vi "DAQmx Run.vi"(11 "Shuwdown Event":refnum<user-event>) -> ()   [LabVIEW 2018, in "Hardware Control.lvlib"]
doc: "<b>Execution System:</b> Data Acquisition"
uses:
  Hardware Control.lvlib
  DAQmx Shortcut.ctl
  Messaging/Message Cluster.ctl
  <vilib>/DAQmx/read.llb/DAQmx Read (Digital 1D Bool NChan 1Samp 1Line).vi
  <vilib>/DAQmx/read.llb/DAQmx Read (Analog 2D DBL NChan NSamp).vi
  <vilib>/Analysis/baseanly.llb/Mean (DBL).vi
  <vilib>/DAQmx/miscellaneous.llb/DAQmx Fill In Error Info.vi
  <vilib>/DAQmx/configure/timing.llb/DAQmx Timing (Sample Clock).vi
  <resource>/objmgr/daqmx.rc
  Messaging/Messaging.lvlib
  <vilib>/Analysis/NI_AALBase.lvlib
panel:
  out "DI Error":errorcluster
  out "AI Error":errorcluster
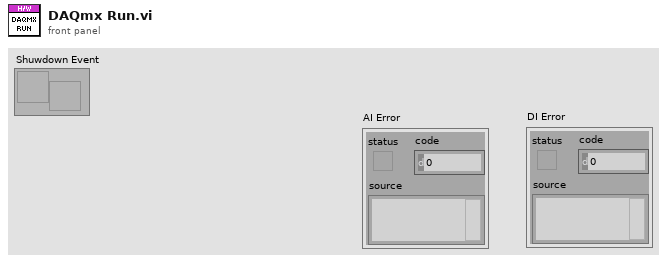
[diagram p1: front panel]
types:
  T1 = typedef "Hardware Control.lvlib/DAQmx Shortcut.ctl" = cluster{"DAQmx Global Channel":refnum<k21>, "Message Queue":string, "Event":string, "Target":string, "Data":variant}
  T2 = typedef "Messaging.lvlib/Message Cluster.ctl" = cluster{"Event":string, "Source":string, "Target":string, "Data":variant}
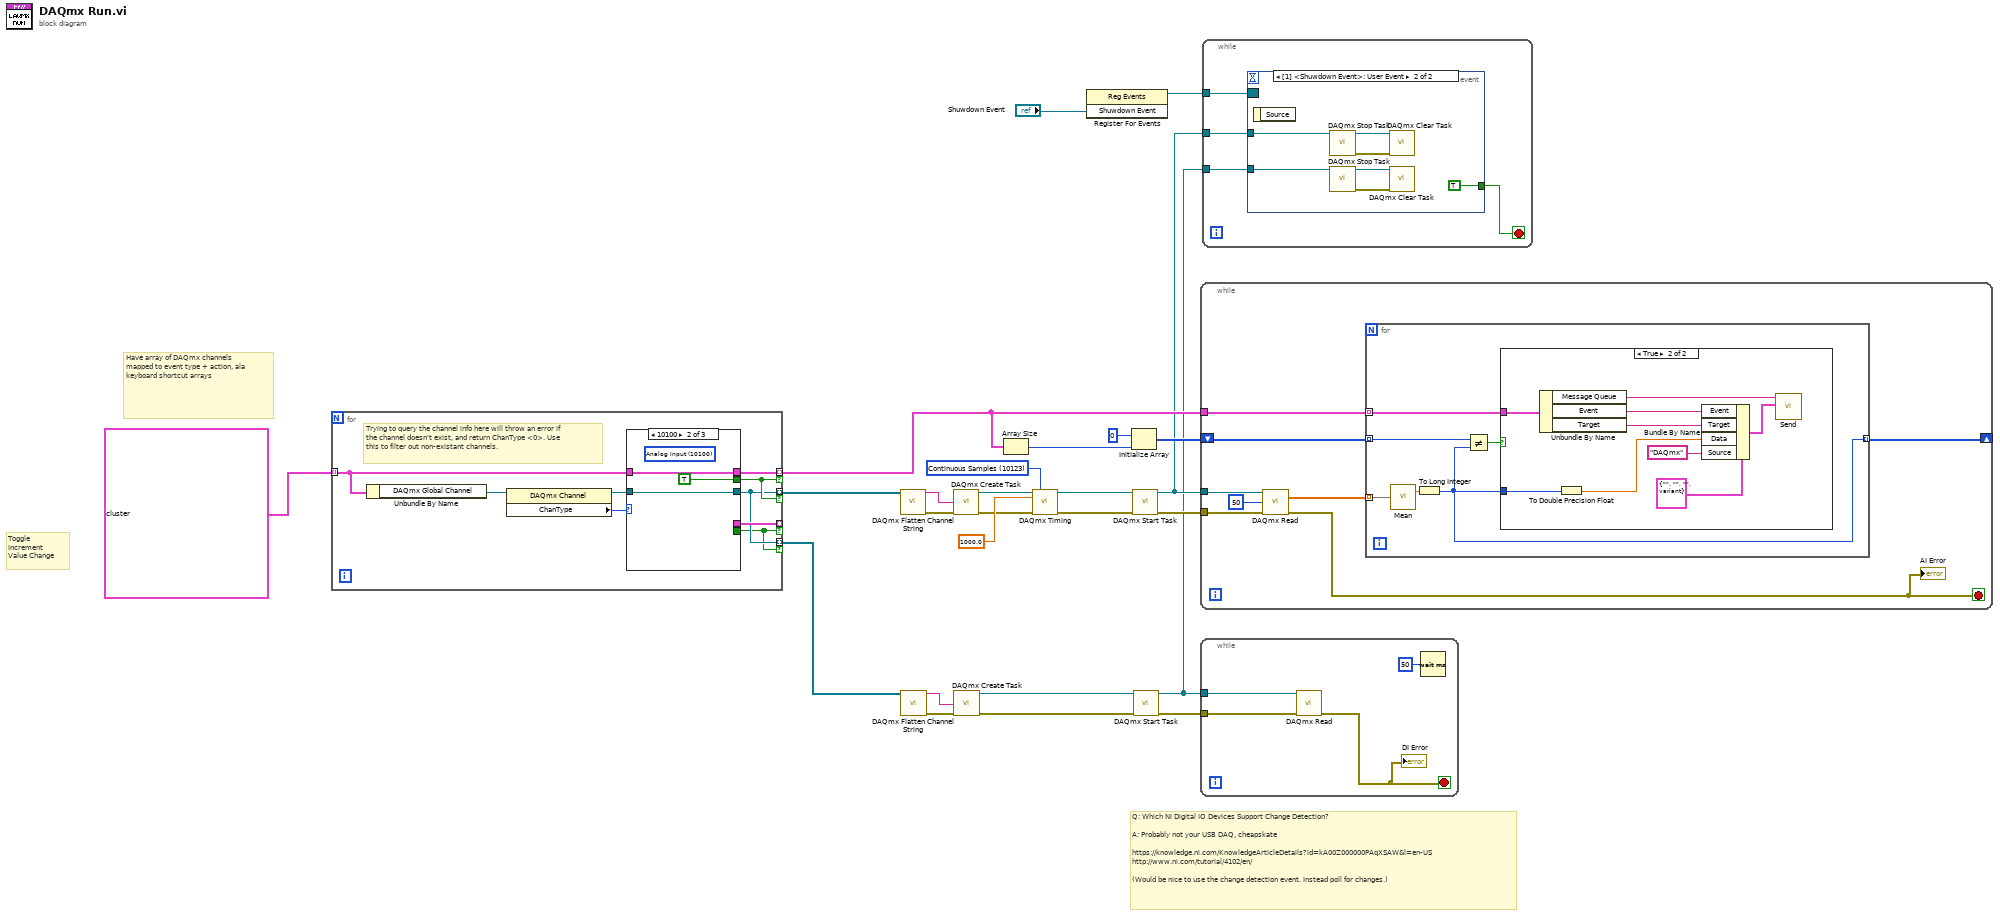
[diagram p0: block diagram]
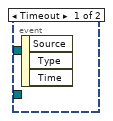
[diagram p2: hidden frame]
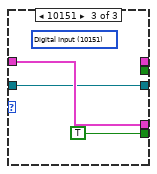
[diagram p5: hidden frame]
diagram:
  w24 = 10123 items=["Finite Samples"=10178, "Continuous Samples"=10123, "Hardware Timed Single Point"=12522] ("sample mode")
  # "Toggle\nIncrement\nValue Change"
  # "Have array of DAQmx channels mapped to event type + action, ala keyboard shortcut arrays"
  # "Q: Which NI Digital IO Devices Support Change Detection?\n\nA: Probably not your USB DAQ, cheapskate\n\nhttps://knowledge.ni.com/KnowledgeArticleDetails?id=kA00Z000000PAqXSAW&l=en-US\nhttp://www.ni.com/tutorial/4102/en/\n\n(Would be nice to use the change detection event. Instead poll for changes.)"
  n1 = for {
    tunnel: T1[] [{"DAQmx Global Channel"="Mixer_Channel1_Level", "Message Queue"="Mixer", "Event"="Value Change", "Target"="Crossfader", "Data"=variant}, {"DAQmx Global Channel"="Deck1_Play", "Message Queue"="Deck1", "Event"="Value Change", "Target"="Play", "Data"=variant}] -> [w32] mode=indexing
    tunnel: [w31] -> w8 mode=indexing if=w28
    tunnel: [w30] -> _ mode=indexing if=w26
    tunnel: [w27] -> w15 mode=indexing if=w28
    tunnel: [w27] -> w12 mode=indexing if=w26
    # "Trying to query the channel info here will throw an error if the channel doesn't exist, and return ChanType <0>. Use this to filter out non-existant channels."
    n2 = Unbundle By Name(w32) -> ("DAQmx Global Channel"=w34:refnum<k21>)
    n3 = property class="DAQmx Channel"(reference=w34) -> (reference out=w29:refnum<k21>, "ChanType"=w33:i32)  [unwired: 1 in, 1 out]
    n4 = case shown="10100" w33 {
      tunnel: w32 -> [_ w37 w40]
      tunnel: [_ w37 _] -> w31
      tunnel: [_ TRUE _] -> w28
      tunnel: [_ _ w40] -> w30
      tunnel: [_ _ TRUE] -> w26
      tunnel: w29 -> [_ w35 w38]
      tunnel: [_ w35 w38] -> w27
      frame Default {
      }
      frame 10100 {
        (unwired) 10100 items=["Analog Input"=10100, "Analog Output"=10102, "Digital Input"=10151, "Digital Output"=10153, "Counter Input"=10131, "Counter Output"=10132] ("ChanType")
      }
      frame 10151 {
        (unwired) 10151 items=["Analog Input"=10100, "Analog Output"=10102, "Digital Input"=10151, "Digital Output"=10153, "Counter Input"=10131, "Counter Output"=10132] ("ChanType")
      }
    }
  }
  n5 = call <vilib>:"DAQmx Flatten Channel String.vi"("names in"=w15) -> ("names out"=w18:string, "error out"=w17:errorcluster)  [unwired: 13 in]
  n6 = call <vilib>:"DAQmx Flatten Channel String.vi"("names in"=w12) -> ("names out"=w13:string, "error out"=w14:errorcluster)  [unwired: 13 in]
  n7 = call <vilib>:"DAQmx Create Task.vi"("global virtual channels"=w18, "error in"=w17) -> ("task out"=w20:refnum<k21>, "error out"=w19:errorcluster)  [unwired: 12 in]
  n8 = call <vilib>:"DAQmx Create Task.vi"("global virtual channels"=w13, "error in"=w14) -> ("task out"=w10:refnum<k21>, "error out"=w9:errorcluster)  [unwired: 12 in]
  n9 = Array Size(array=w8) -> (size(s)=w6:i32)
  n10 = call-poly <vilib>:"DAQmx Timing.vi"("task/channels in"=w20, "sample mode"=w24, "rate"=1000.0, "error in"=w19) -> ("task out"=w23:refnum<k21>, "error out"=w22:errorcluster)  [unwired: 10 in]
  n11 = register-events("Shuwdown Event") -> (reference out=w3:refnum<event-registration>)  [unwired: 2 in, 1 out]
  n12 = Initialize Array(0 ("element"), w6) -> (w5:i32[])
  n13 = call <vilib>:"DAQmx Start Task.vi"("task/channels in"=w23, "error in"=w22) -> ("task out"=w2:refnum<k21>, "error out"=w21:errorcluster)  [unwired: 12 in]
  n14 = call <vilib>:"DAQmx Start Task.vi"("task/channels in"=w10, "error in"=w9) -> ("task out"=w1:refnum<k21>, "error out"=w11:errorcluster)  [unwired: 12 in]
  n15 = while {
    tunnel: w2 -> [w48]
    tunnel: w21 -> [w47]
    tunnel: w8 -> [w43]
    shift-right: [w42] -> _
    shift-left: w5 -> [w44]
    stop <- w41 stop-if-true
    n16 = call-poly <vilib>:"DAQmx Read.vi"("task/channels in"=w48, "number of samples per channel"=50, "error in"=w47) -> ("data"=w45:dbl[][], "error out"=w41:errorcluster)  [unwired: 10 in, 1 out]
    "AI Error" <- w41
    n17 = for {
      tunnel: w45 -> [w54] mode=indexing
      tunnel: w44 -> [w53] mode=indexing
      tunnel: w43 -> [w52] mode=indexing
      tunnel: [w49] -> w42 mode=indexing
      n18 = call-poly <vilib>:"Mean.vi"("X"=w54) -> ("mean"=w50:dbl)  [unwired: 1 out]
      n19 = To Long Integer(number=w50) -> (32bit integer=w49:i32)
      n20 = Not Equal?(x=w53, y=w49) -> (x != y?=w51:bool)
      n21 = case shown="True" w51 {
        tunnel: w52 -> [_ w63]
        tunnel: w49 -> [_ w56]
        frame False {
        }
        frame True {
          n22 = Unbundle By Name(w63) -> ("Message Queue"=w62:string, "Event"=w59:string, "Target"=w58:string)
          n23 = To Double Precision Float(number=w56) -> (double precision float=w55:dbl)
          n24 = Bundle By Name(cluster=T2 {"Event"="", "Source"="", "Target"="", "Data"=variant} ("Message"), "Event"=w59, "Target"=w58, "Data"=w55, "Source"="DAQmx") -> (w60:T2)
          n25 = call "Send.vi"("Message"=w60, "Queue Name"=w62) -> ()  [unwired: 9 in, 1 out]
        }
      }
    }
  }
  n26 = while {
    tunnel: w1 -> [w67]
    tunnel: w11 -> [w66]
    stop <- w64 stop-if-true
    n27 = call-poly <vilib>:"DAQmx Read.vi"("task/channels in"=w67, "error in"=w66) -> ("error out"=w64:errorcluster)  [unwired: 11 in, 2 out]
    "DI Error" <- w64
    n28 = Wait (ms)(milliseconds to wait=u32 50) -> ()  [unwired: 1 out]
  }
  n29 = while {
    tunnel: w3 -> [w71]
    tunnel: w2 -> [w69]
    tunnel: w1 -> [w68]
    stop <- w70 stop-if-true
    n30 = event shown="[1] <Shuwdown Event>: User Event" {
      selector: w71 -> [_ _]
      dyn-events: _ -> [_ _]
      timeout: _ -> [_ _]
      tunnel: [_ TRUE] -> w70
      tunnel: w69 -> [_ w73]
      tunnel: w68 -> [_ w72]
      event Timeout {
        n31 = event-data() -> ()  [unwired: 1 in, 3 out]
      }
      event User Event {
        n32 = event-data() -> ()  [unwired: 1 in, 1 out]
        n33 = call <vilib>:"DAQmx Stop Task.vi"("task/channels in"=w73) -> ("task out"=w76:refnum<k21>, "error out"=w77:errorcluster)  [unwired: 13 in]
        n34 = call <vilib>:"DAQmx Stop Task.vi"("task/channels in"=w72) -> ("task out"=w75:refnum<k21>, "error out"=w74:errorcluster)  [unwired: 13 in]
        n35 = call <vilib>:"DAQmx Clear Task.vi"("task in"=w76, "error in"=w77) -> ()  [unwired: 13 in, 1 out]
        n36 = call <vilib>:"DAQmx Clear Task.vi"("task in"=w75, "error in"=w74) -> ()  [unwired: 13 in, 1 out]
      }
    }
  }
